vi "VIFPGA.vi"(1 "Digital Output":u32, 2 "Enable Digital Output":u32) -> (0 "Digital Input":u32, 3 "Analog Input":i16[](array[numeric]))   [LabVIEW 2012]
uses:
  <vilib>/rvi/eio/common/nirviEmuTemplateMethod_errors.vi
  <vilib>/eio/EIOMethodNode/EIOMethodNode.xnode
  <vilib>/eio/EIONode/EIONode.xnode
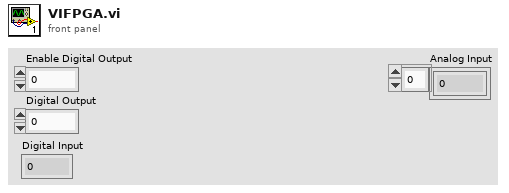
[diagram p1: front panel]
types:
  T1 = cluster{"Mod1/AI0":i16, "Mod1/AI1":i16, "Mod1/AI2":i16, "Mod1/AI3":i16}
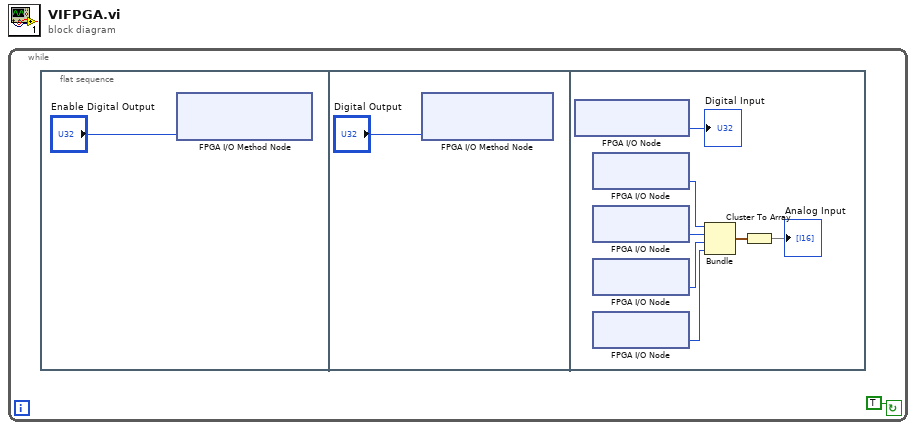
[diagram p0: block diagram]
diagram:
  n1 = while {
    stop <- TRUE continue-if-true
    n2 = flat-sequence {
      frame #0 {
        n3 = xnode "FPGA I/O Method Node"("Enable"="Enable Digital Output") -> ()  [unwired: 1 in, 1 out]
      }
      frame #1 {
        n4 = xnode "FPGA I/O Method Node"("Data"="Digital Output") -> ()  [unwired: 1 in, 1 out]
      }
      frame #2 {
        n5 = xnode "FPGA I/O Node"() -> ("Mod2/DIO7:0"=→"Digital Input":u8)  [unwired: 1 in, 1 out]
        n6 = xnode "FPGA I/O Node"() -> ("Mod1/AI0"=w4:i16)  [unwired: 1 in, 1 out]
        n7 = xnode "FPGA I/O Node"() -> ("Mod1/AI1"=w5:i16)  [unwired: 1 in, 1 out]
        n8 = xnode "FPGA I/O Node"() -> ("Mod1/AI2"=w6:i16)  [unwired: 1 in, 1 out]
        n9 = xnode "FPGA I/O Node"() -> ("Mod1/AI3"=w7:i16)  [unwired: 1 in, 1 out]
        n10 = Bundle("Mod1/AI0"=w4, "Mod1/AI1"=w5, "Mod1/AI2"=w6, "Mod1/AI3"=w7) -> (w8:T1)  [unwired: 1 in]
        n11 = Cluster To Array(cluster=w8) -> (array=→"Analog Input":i16[])
      }
    }
  }
